vi "Charging State Color.vi"(4 "error in":errorcluster, 7 "Str Refnum":refnum<vi>) -> (0 "error out":errorcluster)   [LabVIEW 2010]
panel:
  in  "Labels":string[](array[string])=["default", "CHARGE_OFF-0", "CHARGE_PRE_CONDITION-1", "CHARGE_CC_FAST-2", "CHARGE_CC_SLOW-3", "CHARGE_COMPLETE-4", "CHARGE_ERROR-5"]
  in  "BG":u32[](array[colorbox])=[16448250, 8454143, 16777238, 16744512, 16635906, 6618880, 16711680]
  # "Prerequisites:\nChange the Referenced String color to Transparent [T]."
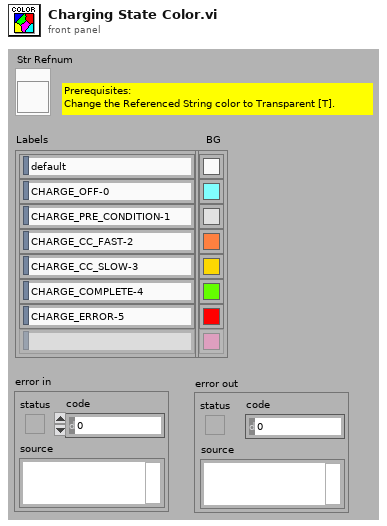
[diagram p1: front panel]
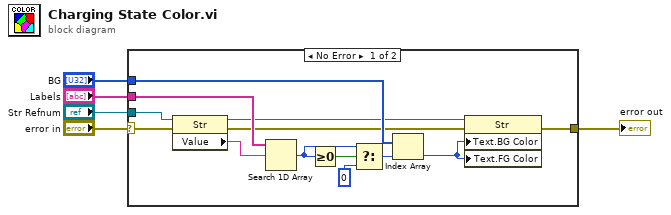
[diagram p0: block diagram]
diagram:
  n1 = case shown="No Error" "error in" {
    selector: "error in" -> [w8 w19]
    tunnel: "BG" -> [w18 _]
    tunnel: "Labels" -> [w17 _]
    tunnel: [w16 w19] -> w3
    tunnel: "Str Refnum" -> [w9 _]
    frame No Error {
      n2 = property class="Str"(reference=w9, error in=w8) -> (reference out=w7:refnum<vi>, error out=w12:errorcluster, "Value"=w11:string)
      n3 = Search 1D Array(1D array=w17, element=w11) -> (index of element=w10:i32)  [unwired: 1 in]
      n4 = Greater Or Equal To 0?(x=w10) -> (x >= 0?=w15:bool)
      n5 = Select(t=w10, s=w15, f=0) -> (s? t:f=w13:i32)
      n6 = Index Array(array=w18, index=w13) -> (element=w6:u32)
      n7 = property class="Str"(reference=w7, error in=w12, "Text.BG Color"=w6, "Text.FG Color"=w6) -> (error out=w16:errorcluster)  [unwired: 1 out]
    }
    frame Error {
    }
  }
  "error out" <- w3
